vi "FGV_Position_Table.vi"(3 "error in":errorcluster, 4 "Position table":dbl[][](array[numeric]), 5 "Action":T1) -> (0 "error out":errorcluster, 1 "Position table":dbl[][](array[numeric]), 2 "N pos":i32)   [LabVIEW 2026]
uses:
  Controls/TypeDef_FGV.ctl
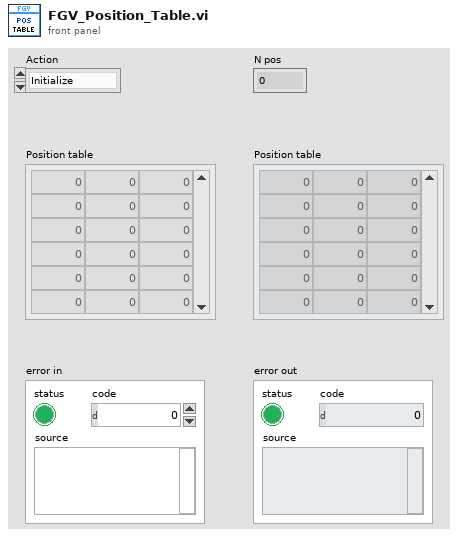
[diagram p1: front panel]
types:
  T1 = typedef "TypeDef_FGV.ctl" = enum16{"Initialize", "Write", "Read"}
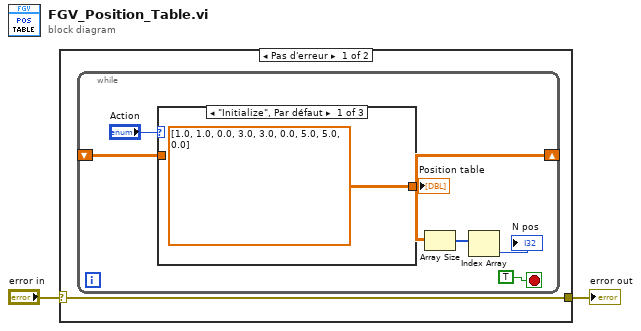
[diagram p0: block diagram]
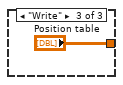
[diagram p3: hidden frame]
diagram:
  n1 = case shown="Pas d'erreur" "error in" {
    selector: "error in" -> [w3 w13]
    tunnel: [w3 w13] -> w2
    frame No Error {
      n2 = while {
        shift-right: [w5] -> _
        shift-left: _ -> [w7]
        stop <- TRUE stop-if-true
        n3 = case shown="\"Initialize\", Par défaut" "Action" {
          tunnel: [dbl[][] [[1.0, 1.0, 0.0], [3.0, 3.0, 0.0], [5.0, 5.0, 0.0]] ("Tableau - Numérique") w11 "Position table"] -> w5
          tunnel: w7 -> [_ w11 _]
          frame "Initialize", Default {
          }
          frame "Read" {
          }
          frame "Write" {
          }
        }
        "Position table" <- w5
        n4 = Array Size(array=w5) -> (size(s)=w6:i32[])
        n5 = Index Array(array=w6) -> (element=→"N pos":i32)  [unwired: 1 in]
      }
    }
    frame Error {
    }
  }
  "error out" <- w2
